vi "Variant to String.vi"(8 "error in (no error)":errorcluster, 10 "Variant":variant, 11 "StringFormatter in":refnum<class "StringFormatter.lvclass">) -> (0 "error out":errorcluster, 2 "Value":string, 3 "StringFormatter out":refnum<class "StringFormatter.lvclass">)   [LabVIEW 2013, in "OpenStringFormatter.lvlib" / "StringFormatter.lvclass"]
uses:
  StringFormatter.lvclass
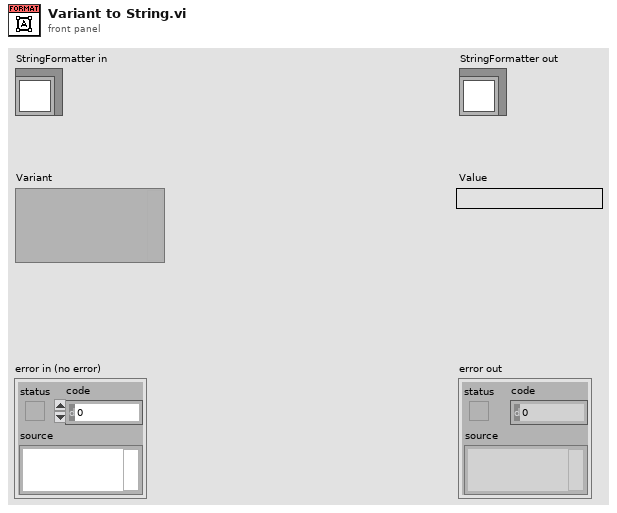
[diagram p1: front panel]
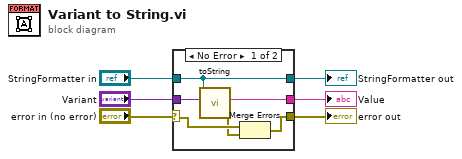
[diagram p0: block diagram]
diagram:
  n1 = case shown="No Error" "error in (no error)" {
    selector: "error in (no error)" -> [w9 w14]
    tunnel: [w7 w14] -> w5
    tunnel: [w10 w13] -> w3
    tunnel: "StringFormatter in" -> [w10 w13]
    tunnel: "Variant" -> [w12 _]
    tunnel: [w11 _] -> w1
    frame No Error {
      n2 = call-dynamic "toString.vi"("Variant"=w12, "StringFormatter in"=w10) -> ("error out"=w8:errorcluster, "Value"=w11:string)  [unwired: 8 in]
      n3 = Merge Errors(w9, w8) -> (w7:errorcluster)
    }
    frame Error {
    }
  }
  "error out" <- w5
  "StringFormatter out" <- w3
  "Value" <- w1
